vi "LDA_Vel_max_min.vi"(1 "Multiply Velocity by -1":bool, 3 "Centre Velocity":u16(ring)=16 items=["0.000E+0", "0.000E+0", "0.000E+0", "0.000E+0", "0.000E+0", "0.000E+0", "0.000E+0", "0.000E+0", "0.000E+0", "0.000E+0", "0.000E+0", "0.000E+0"], 4 "Velocity span":u16(ring)=10 items=["976.562E+0", "1.953E+3", "3.906E+3", "7.812E+3", "15.625E+3", "31.250E+3", "62.500E+3", "125.000E+3", "250.000E+3", "500.000E+3", "1.000E+6", "2.000E+6", "4.000E+6", "8.000E+6"], 5 "Centres":dbl[](array[numeric]), 6 "Spans":dbl[](array[numeric])) -> (0 "Selected range":cluster{"Minimum":dbl, "Maximum":dbl}={"Minimum"=-1.9850000000000005, "Maximum"=1.9850000000000005} {"Maximum" format="%.2f"; "Minimum" format="%.2f"})   [LabVIEW 2011]
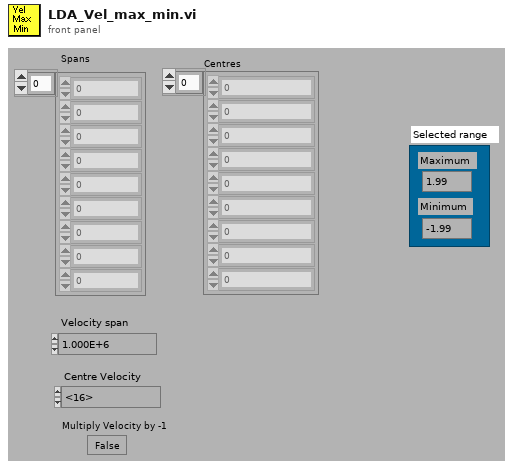
[diagram p1: front panel]
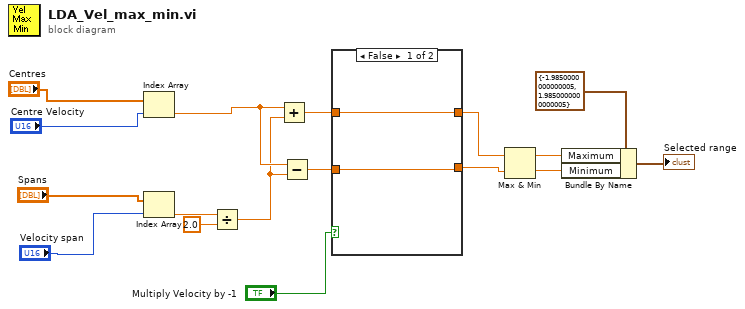
[diagram p0: block diagram]
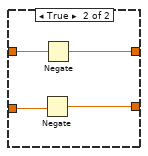
[diagram p2: hidden frame]
diagram:
  n1 = Index Array(array="Centres", index="Centre Velocity") -> (element=w11:dbl)
  n2 = Index Array(array="Spans", index="Velocity span") -> (element=w13:dbl)
  n3 = Divide(x=w13, y=2.0) -> (x/y=w10:dbl)
  n4 = Add(x=w11, y=w10) -> (x+y=w8:dbl)
  n5 = Subtract(x=w11, y=w10) -> (x-y=w7:dbl)
  n6 = case shown="False" "Multiply Velocity by -1" {
    tunnel: w8 -> [w19 w23]
    tunnel: w7 -> [w18 w22]
    tunnel: [w19 w21] -> w2
    tunnel: [w18 w20] -> w1
    frame False {
    }
    frame True {
      n7 = Negate(x=w22) -> (-x=w20:dbl)
      n8 = Negate(x=w23) -> (-x=w21:dbl)
    }
  }
  n9 = Max & Min(x=w2, y=w1) -> (max(x,y)=w4:dbl, min(x,y)=w3:dbl)
  n10 = Bundle By Name(cluster=cluster{"Minimum":dbl, "Maximum":dbl} {"Minimum"=-1.9850000000000005, "Maximum"=1.9850000000000005} ("Selected range"), "Maximum"=w4, "Minimum"=w3) -> (→"Selected range":cluster{"Minimum":dbl, "Maximum":dbl})
